vi "Publish ILC Inputs.vi"(8 "error in (no error)":errorcluster, 11 "Model in":refnum<class "Model.lvclass">) -> (0 "error out":errorcluster, 3 "Model out":refnum<class "Model.lvclass">)   [LabVIEW 2015, in "Model.lvclass"]
uses:
  Model.lvclass
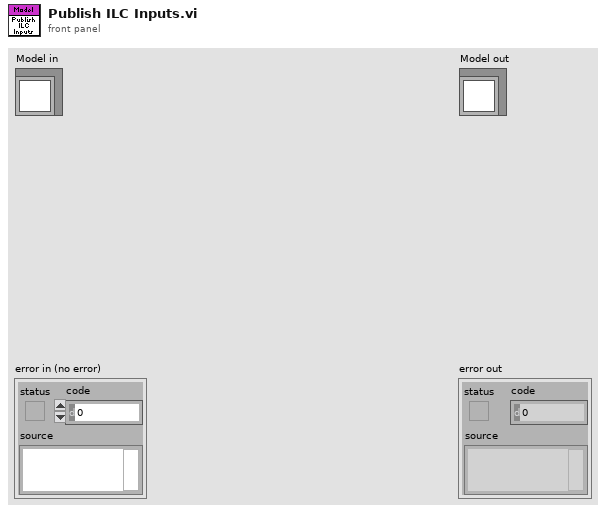
[diagram p1: front panel]
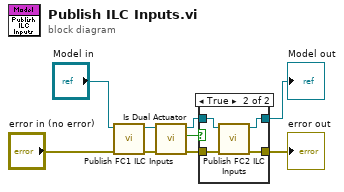
[diagram p0: block diagram]
diagram:
  n1 = call "Publish FC1 ILC Inputs.vi"("error in (no error)"="error in (no error)", "Model in"="Model in") -> ("error out"=w3:errorcluster, "Model out"=w2:refnum<class "Model.lvclass">)  [unwired: 8 in]
  n2 = call "Is Dual Actuator.vi"("error in (no error)"=w3, "Model in"=w2) -> ("error out"=w7:errorcluster, "Is Dual Actuator"=w9:bool, "Model out"=w8:refnum<class "Model.lvclass">)  [unwired: 7 in]
  n3 = case shown="True" w9 {
    tunnel: w8 -> [w11 w15]
    tunnel: w7 -> [w10 w14]
    tunnel: [w10 w13] -> w5
    tunnel: [w11 w12] -> w6
    frame False {
    }
    frame True {
      n4 = call "Publish FC2 ILC Inputs.vi"("error in (no error)"=w14, "Model in"=w15) -> ("error out"=w13:errorcluster, "Model out"=w12:refnum<class "Model.lvclass">)  [unwired: 8 in]
    }
  }
  "error out" <- w5
  "Model out" <- w6
